vi "Calculate angle.vi"(9 "Mouse release coordinates":cluster{"X":sgl, "Y":sgl}, 10 "Circle":T1, 11 "Angle (in degrees)":dbl format="%#_13g") -> (3 "Angle":dbl)   [LabVIEW 2019]
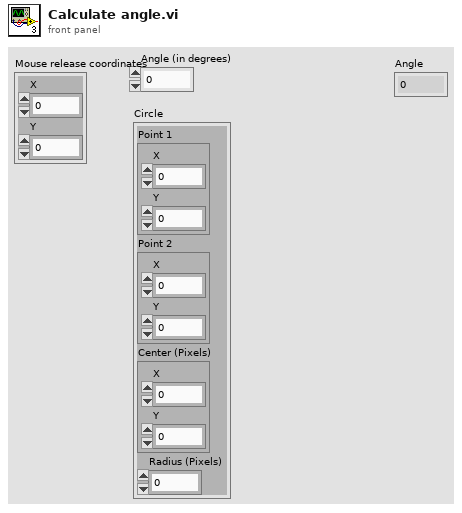
[diagram p1: front panel]
types:
  T1 = cluster{"Point 1":cluster{"X":sgl, "Y":sgl}, "Point 2":cluster{"X":sgl, "Y":sgl}, "Center (Pixels)":cluster{"X":sgl, "Y":sgl}, "Radius (Pixels)":dbl}
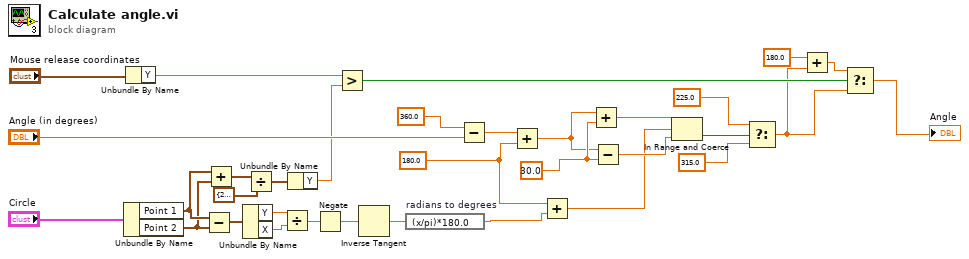
[diagram p0: block diagram]
diagram:
  w24 = sgl 30.0 ("y")
  w15 = sgl 180.0 ("y")
  n1 = Unbundle By Name("Circle") -> ("Point 1"=w12:cluster{"X":sgl, "Y":sgl}, "Point 2"=w11:cluster{"X":sgl, "Y":sgl})
  n2 = Unbundle By Name("Mouse release coordinates") -> ("Y"=w7:sgl)
  n3 = Subtract(x=w12, y=w11) -> (x-y=w32:cluster{"X":sgl, "Y":sgl})
  n4 = Add(x=w12, y=w11) -> (x+y=w10:cluster{"X":sgl, "Y":sgl})
  n5 = Unbundle By Name(w32) -> ("Y"=w31:sgl, "X"=w30:sgl)
  n6 = Divide(x=w10, y=cluster{"X":sgl, "Y":sgl} {"X"=2.0, "Y"=2.0}) -> (x/y=w8:cluster{"X":sgl, "Y":sgl})
  n7 = Divide(x=w31, y=w30) -> (x/y=w28:sgl)
  n8 = Unbundle By Name(w8) -> ("Y"=w6:sgl)
  n9 = Negate(x=w28) -> (-x=w27:sgl)
  n10 = Greater?(x=w7, y=w6) -> (0:w5:bool)
  n11 = Inverse Tangent(1:w27) -> (0:w29:sgl)
  n12 = expression code="(x/pi)*180.0" "radians to degrees"(w29) -> (w16:sgl)
  n13 = Subtract(x=sgl 360.0, y="Angle (in degrees)") -> (x-y=w25:dbl)
  n14 = Add(x=w25, y=w15) -> (x+y=w21:dbl)
  n15 = Add(x=w15, y=w16) -> (x+y=w14:sgl)
  n16 = Add(x=w21, y=w24) -> (x+y=w20:dbl)
  n17 = Subtract(x=w21, y=w24) -> (x-y=w22:dbl)
  n18 = In Range and Coerce(upper limit=w20, x=w14, lower limit=w22) -> (In Range?=w19:bool)  [unwired: 1 out]
  n19 = Select(t=225.0, s=w19, f=315.0) -> (s? t:f=w4:dbl)
  n20 = Add(x=180.0, y=w4) -> (x+y=w2:dbl)
  n21 = Select(t=w2, s=w5, f=w4) -> (s? t:f=→"Angle":dbl)
